vi "Pressure 2016.vi"(2 "Zero Pressure\n(F = leave as is)":bool, 3 "Pressure Offset":dbl format="%.2f") -> (1 "Pressure":dbl format="%.2f")   [LabVIEW 2016]
uses:
  KPRO_lv2015/Kpro Globals.vi
panel:
  out "Voltage":dbl format="%.2f"
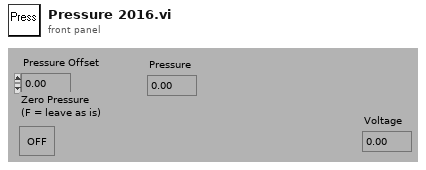
[diagram p1: front panel]
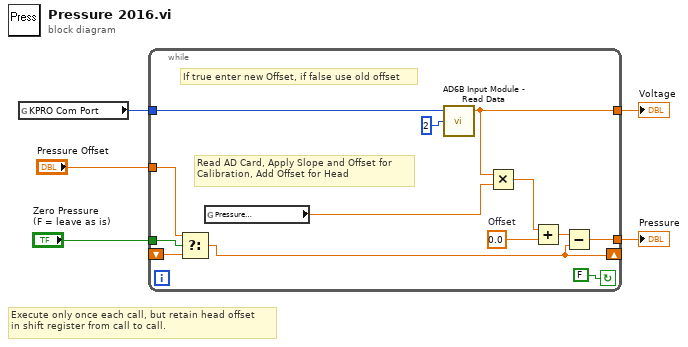
[diagram p0: block diagram]
diagram:
  # "Execute only once each call, but retain head offset \nin shift register from call to call."
  n1 = global read "Kpro Globals.vi" "KPRO Com Port"() -> (w2:i32)
  n2 = while {
    tunnel: "Zero Pressure\n(F = leave as is)" -> [w13]
    tunnel: "Pressure Offset" -> [w14]
    shift-left: _ -> [w15]
    shift-right: [w9] -> _
    tunnel: [w12] -> w5
    tunnel: w2 -> [w8]
    tunnel: [w6] -> w1
    stop <- FALSE continue-if-true
    w16 = 0.0  # Offset
    # "Read AD Card, Apply Slope and Offset for\nCalibration, Add Offset for Head"
    # "If true enter new Offset, if false use old offset"
    n3 = Select(t=w14, s=w13, f=w15) -> (s? t:f=w9:dbl)
    n4 = global read "Kpro Globals.vi" "Pressure \nSlope"() -> (w7:dbl)
    n5 = call "AD6B Input Module - Read Data.VI"("address (0 to 255)"=2, "port number (1:com2)"=w8) -> ("scaled data"=w6:dbl)  [unwired: 1 in, 2 out]
    n6 = Multiply(x=w6, y=w7) -> (x*y=w17:dbl)
    n7 = Add(x=w17, y=w16) -> (x+y=w10:dbl)
    n8 = Subtract(x=w10, y=w9) -> (x-y=w12:dbl)
  }
  "Pressure" <- w5
  "Voltage" <- w1
